vi "globalprogram testen.vi"() -> (2 "Array 2":i32[](array[numeric]), 3 "Numeric 2":i32)   [LabVIEW 2019]
uses:
  <vilib>/myRIO/Common/Instrument Driver Framework/Utilities/typedefs/Analog Scaling Constants.ctl
  <vilib>/myRIO/Common/Instrument Driver Framework/Utilities/typedefs/Analog Scaling Constants List.ctl
  <vilib>/myRIO/Common/Instrument Driver Framework/myRIO v1.0/AO/typedefs/AO Channels Enum.ctl
  <vilib>/myRIO/Common/Instrument Driver Framework/myRIO v1.0/AO/typedefs/AO Channels List.ctl
  <vilib>/myRIO/Common/Instrument Driver Framework/Utilities/typedefs/Generic FPGA Reference.ctl
  <vilib>/myRIO/Common/Instrument Driver Framework/Utilities/typedefs/myRIO v1.0 Reference.ctl
  <vilib>/myRIO/Common/Instrument Driver Framework/Utilities/typedefs/Hardware Version Enum.ctl
  <vilib>/myRIO/Common/Instrument Driver Framework/Utilities/typedefs/myRIO Generic Hardware Reference.ctl
  <vilib>/myRIO/Instrument Drivers/Onboard IO/AO/typedefs/AO Reference.ctl
  <vilib>/myRIO/Instrument Drivers/Onboard IO/AO/AO.lvlib
  <vilib>/myRIO/Instrument Drivers/Onboard IO/AO/vis/Write.vi
  <vilib>/userDefined/High Color/nirio_resource_hc.ctl
  <vilib>/myRIO/Common/Instrument Driver Framework/myRIO v1.0/AO/vis/myRIO v1.1 Open AO.vi
  <vilib>/myRIO/Instrument Drivers/Onboard IO/AO/vis/myRIO AO Open.xnode
  <vilib>/myRIO/Common/Instrument Driver Framework/Utilities/vis/Is FPGA Ref Available.vi
  <vilib>/myRIO/Express VI/Onboard IO/AO/AO Express VI.xnode
  <vilib>/myRIO/Common/Instrument Driver Framework/myRIO v1.0/DIO/typedefs/DIO Channels Enum.ctl
  <vilib>/myRIO/Common/Instrument Driver Framework/myRIO v1.0/DIO/typedefs/DIO Channels List.ctl
  <vilib>/myRIO/Instrument Drivers/Onboard IO/DIO/typedefs/DIO Reference.ctl
  <vilib>/myRIO/Instrument Drivers/Onboard IO/DIO/DIO.lvlib
  <vilib>/myRIO/Instrument Drivers/Onboard IO/DIO/vis/myRIO DIO Open.xnode
  <vilib>/myRIO/Common/Instrument Driver Framework/myRIO v1.0/DIO/vis/myRIO v1.1 Open DIO.vi
  <vilib>/myRIO/Instrument Drivers/Onboard IO/DIO/vis/Write.vi
  <vilib>/myRIO/Express VI/Onboard IO/DO/DO Express VI.xnode
  <vilib>/myRIO/Express VI/Onboard IO/DI/DI Express VI.xnode
  <vilib>/myRIO/Instrument Drivers/Onboard IO/DIO/vis/Read.vi
  Global.vi
  <vilib>/myRIO/Express VI/Onboard IO/AI/AI Express VI.xnode
  <vilib>/myRIO/Instrument Drivers/Onboard IO/AI/typedefs/AI Reference.ctl
  <vilib>/myRIO/Instrument Drivers/Onboard IO/AI/AI.lvlib
  <vilib>/myRIO/Common/Instrument Driver Framework/myRIO v1.0/AI/typedefs/AI Channels List.ctl
  <vilib>/myRIO/Common/Instrument Driver Framework/myRIO v1.0/AI/typedefs/AI Channels Enum.ctl
  <vilib>/myRIO/Instrument Drivers/Onboard IO/AI/vis/Read.vi
  <vilib>/myRIO/Instrument Drivers/Onboard IO/AI/vis/myRIO AI Open.xnode
  <vilib>/myRIO/Common/Instrument Driver Framework/myRIO v1.0/AI/vis/myRIO v1.1 Open AI.vi
panel:
  in  "MANUEEL":bool
  in  "STOP":bool
  in  "tijdsinterval 8":dbl
  in  "tijdsinterval 7":dbl
  in  "tijdsinterval 6":dbl
  in  "tijdsinterval 5":dbl
  in  "tijdsinterval 4":dbl
  in  "tijdsinterval 3":dbl
  in  "tijdsinterval 2":dbl
  out "A/DIO1 (Pin 13)":bool
  in  "stoppen":bool
  in  "rechts draaien achteruit":bool
  in  "links draaien achteruit":bool
  out "appended array":dbl[](array[numeric])
  in  "snelheid":dbl
  in  "rechts draaien":bool
  in  "links draaien":bool
  in  "achterwaarts":bool
  in  "voorwaarts":bool
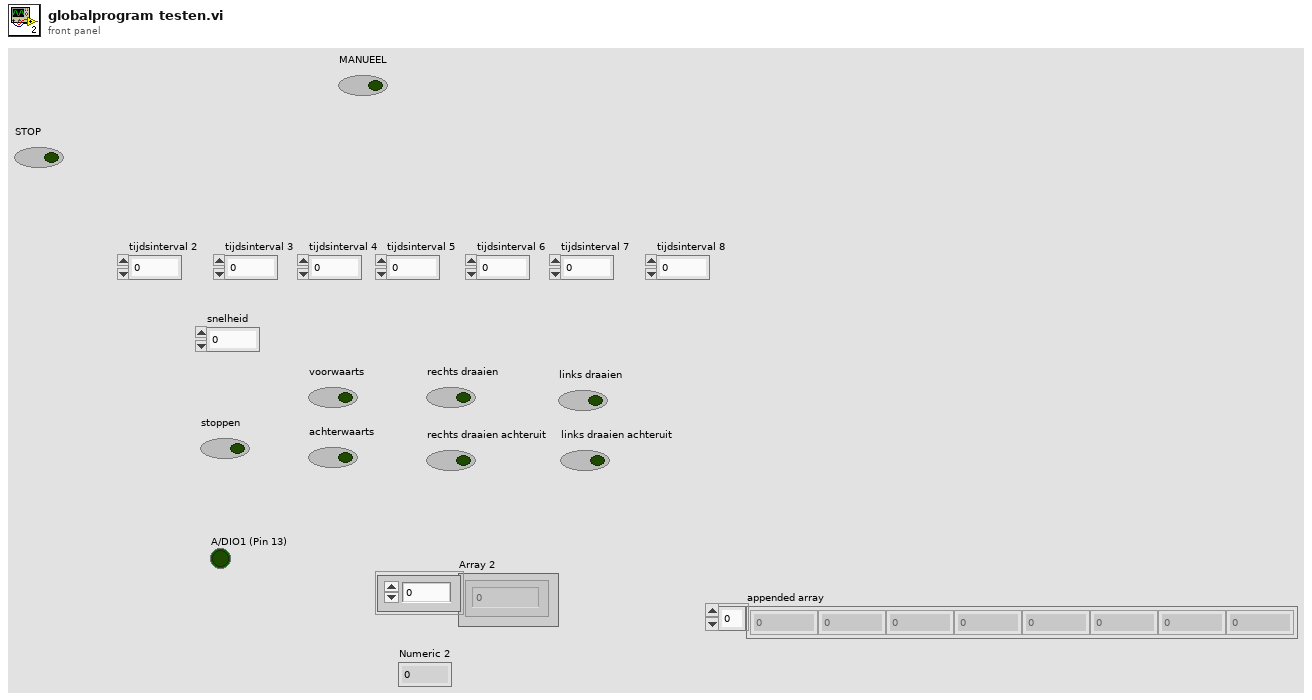
[diagram p1: front panel]
types:
  T1 = typedef "DIO.lvlib/DIO Reference.ctl" = cluster{"myRIO Reference":T2, "DIO Channels List":T6}
  T2 = typedef "myRIO Generic Hardware Reference.ctl" = cluster{"myRIO Model":T3, "myRIO Hardware Reference":T4}
  T3 = typedef "Hardware Version Enum.ctl" = enum16{"Unknown", "myRIO-1900", "myRIO-1950", "roboRIO", "NI ELVIS RIO CM", "ELVIS III"}
  T4 = typedef "myRIO v1.0 Reference.ctl" = cluster{"Generic FPGA Reference":T5, "Allow multiple opens":bool}
  T5 = typedef "Generic FPGA Reference.ctl" = refnum<k20>
  T6 = typedef "DIO Channels List.ctl" = T7[]
  T7 = typedef "DIO Channels Enum.ctl" = enum16{"Not Connected", "C/DIO0", "C/DIO1", "C/DIO2", "C/DIO3", "C/DIO4", "C/DIO5", "C/DIO6", "C/DIO7", "A/DIO0", "A/DIO1", "A/DIO2", "A/DIO3", "A/DIO4", "A/DIO5", "A/DIO6", "A/DIO7", "A/DIO8", "A/DIO9", "A/DIO10", "A/DIO11", "A/DIO12", "A/DIO13", "A/DIO14", "A/DIO15", "A/DIO16", "A/DIO17", "A/DIO18", "A/DIO19", "B/DIO0", "B/DIO1", "B/DIO2", "B/DIO3", "B/DIO4", "B/DIO5", "B/DIO6", "B/DIO7", "B/DIO8", "B/DIO9", "B/DIO10", "B/DIO11", "B/DIO12", "B/DIO13", "B/DIO14", "B/DIO15", "B/DIO16", "B/DIO17", "B/DIO18", "B/DIO19", "LED0", "LED1", "LED2", "LED3", "Button0", "DIO/DIO0", "DIO/DIO1", "DIO/DIO2", "DIO/DIO3", "DIO/DIO4", "DIO/DIO5", "DIO/DIO6", "DIO/DIO7", "DIO/DIO8", "DIO/DIO9", "SPI/CS0", "SPI/CS1", "SPI/CS2", "SPI/CS3", "LED RADIO (Green)", "LED RADIO (Red)", "LED COMM (Green)", "LED COMM (Red)", "LED MODE (Green)", "LED MODE (Red)"}
  T8 = typedef "nirio_resource_hc.ctl" = tag
  T9 = typedef "AO.lvlib/AO Reference.ctl" = cluster{"myRIO Reference":T2, "AO Channel List":T10, "AO Scaling Constant List":T12}
  T10 = typedef "AO Channels List.ctl" = T11[]
  T11 = typedef "AO Channels Enum.ctl" = enum16{"Not Connected", "AudioOut/Left", "AudioOut/Right", "C/AO0", "C/AO1", "A/AO0", "A/AO1", "B/AO0", "B/AO1"}
  T12 = typedef "Analog Scaling Constants List.ctl" = T13[]
  T13 = typedef "Analog Scaling Constants.ctl" = cluster{"LSB Weight (Volts)":dbl, "Offset (Volts)":dbl, "Signed?":bool}
  T14 = typedef "AI.lvlib/AI Reference.ctl" = cluster{"myRIO Reference":T2, "AI Channels List":T15, "AI Scaling Constants List":T12}
  T15 = typedef "AI Channels List.ctl" = T16[]
  T16 = typedef "AI Channels Enum.ctl" = enum16{"Not Connected", "AudioIn/Left", "AudioIn/Right", "C/AI0", "C/AI1", "A/AI0", "A/AI1", "A/AI2", "A/AI3", "A/AI4", "A/AI5", "A/AI6", "A/AI7", "B/AI0", "B/AI1", "B/AI2", "B/AI3", "B/AI4", "B/AI5", "B/AI6", "B/AI7", "AI/AI0", "AI/AI1", "AI/AI2", "AI/AI3", "A/AI0 (DIFF)", "A/AI1 (DIFF)", "A/AI2 (DIFF)", "A/AI3 (DIFF)", "B/AI0 (DIFF)", "B/AI1 (DIFF)", "B/AI2 (DIFF)", "B/AI3 (DIFF)"}
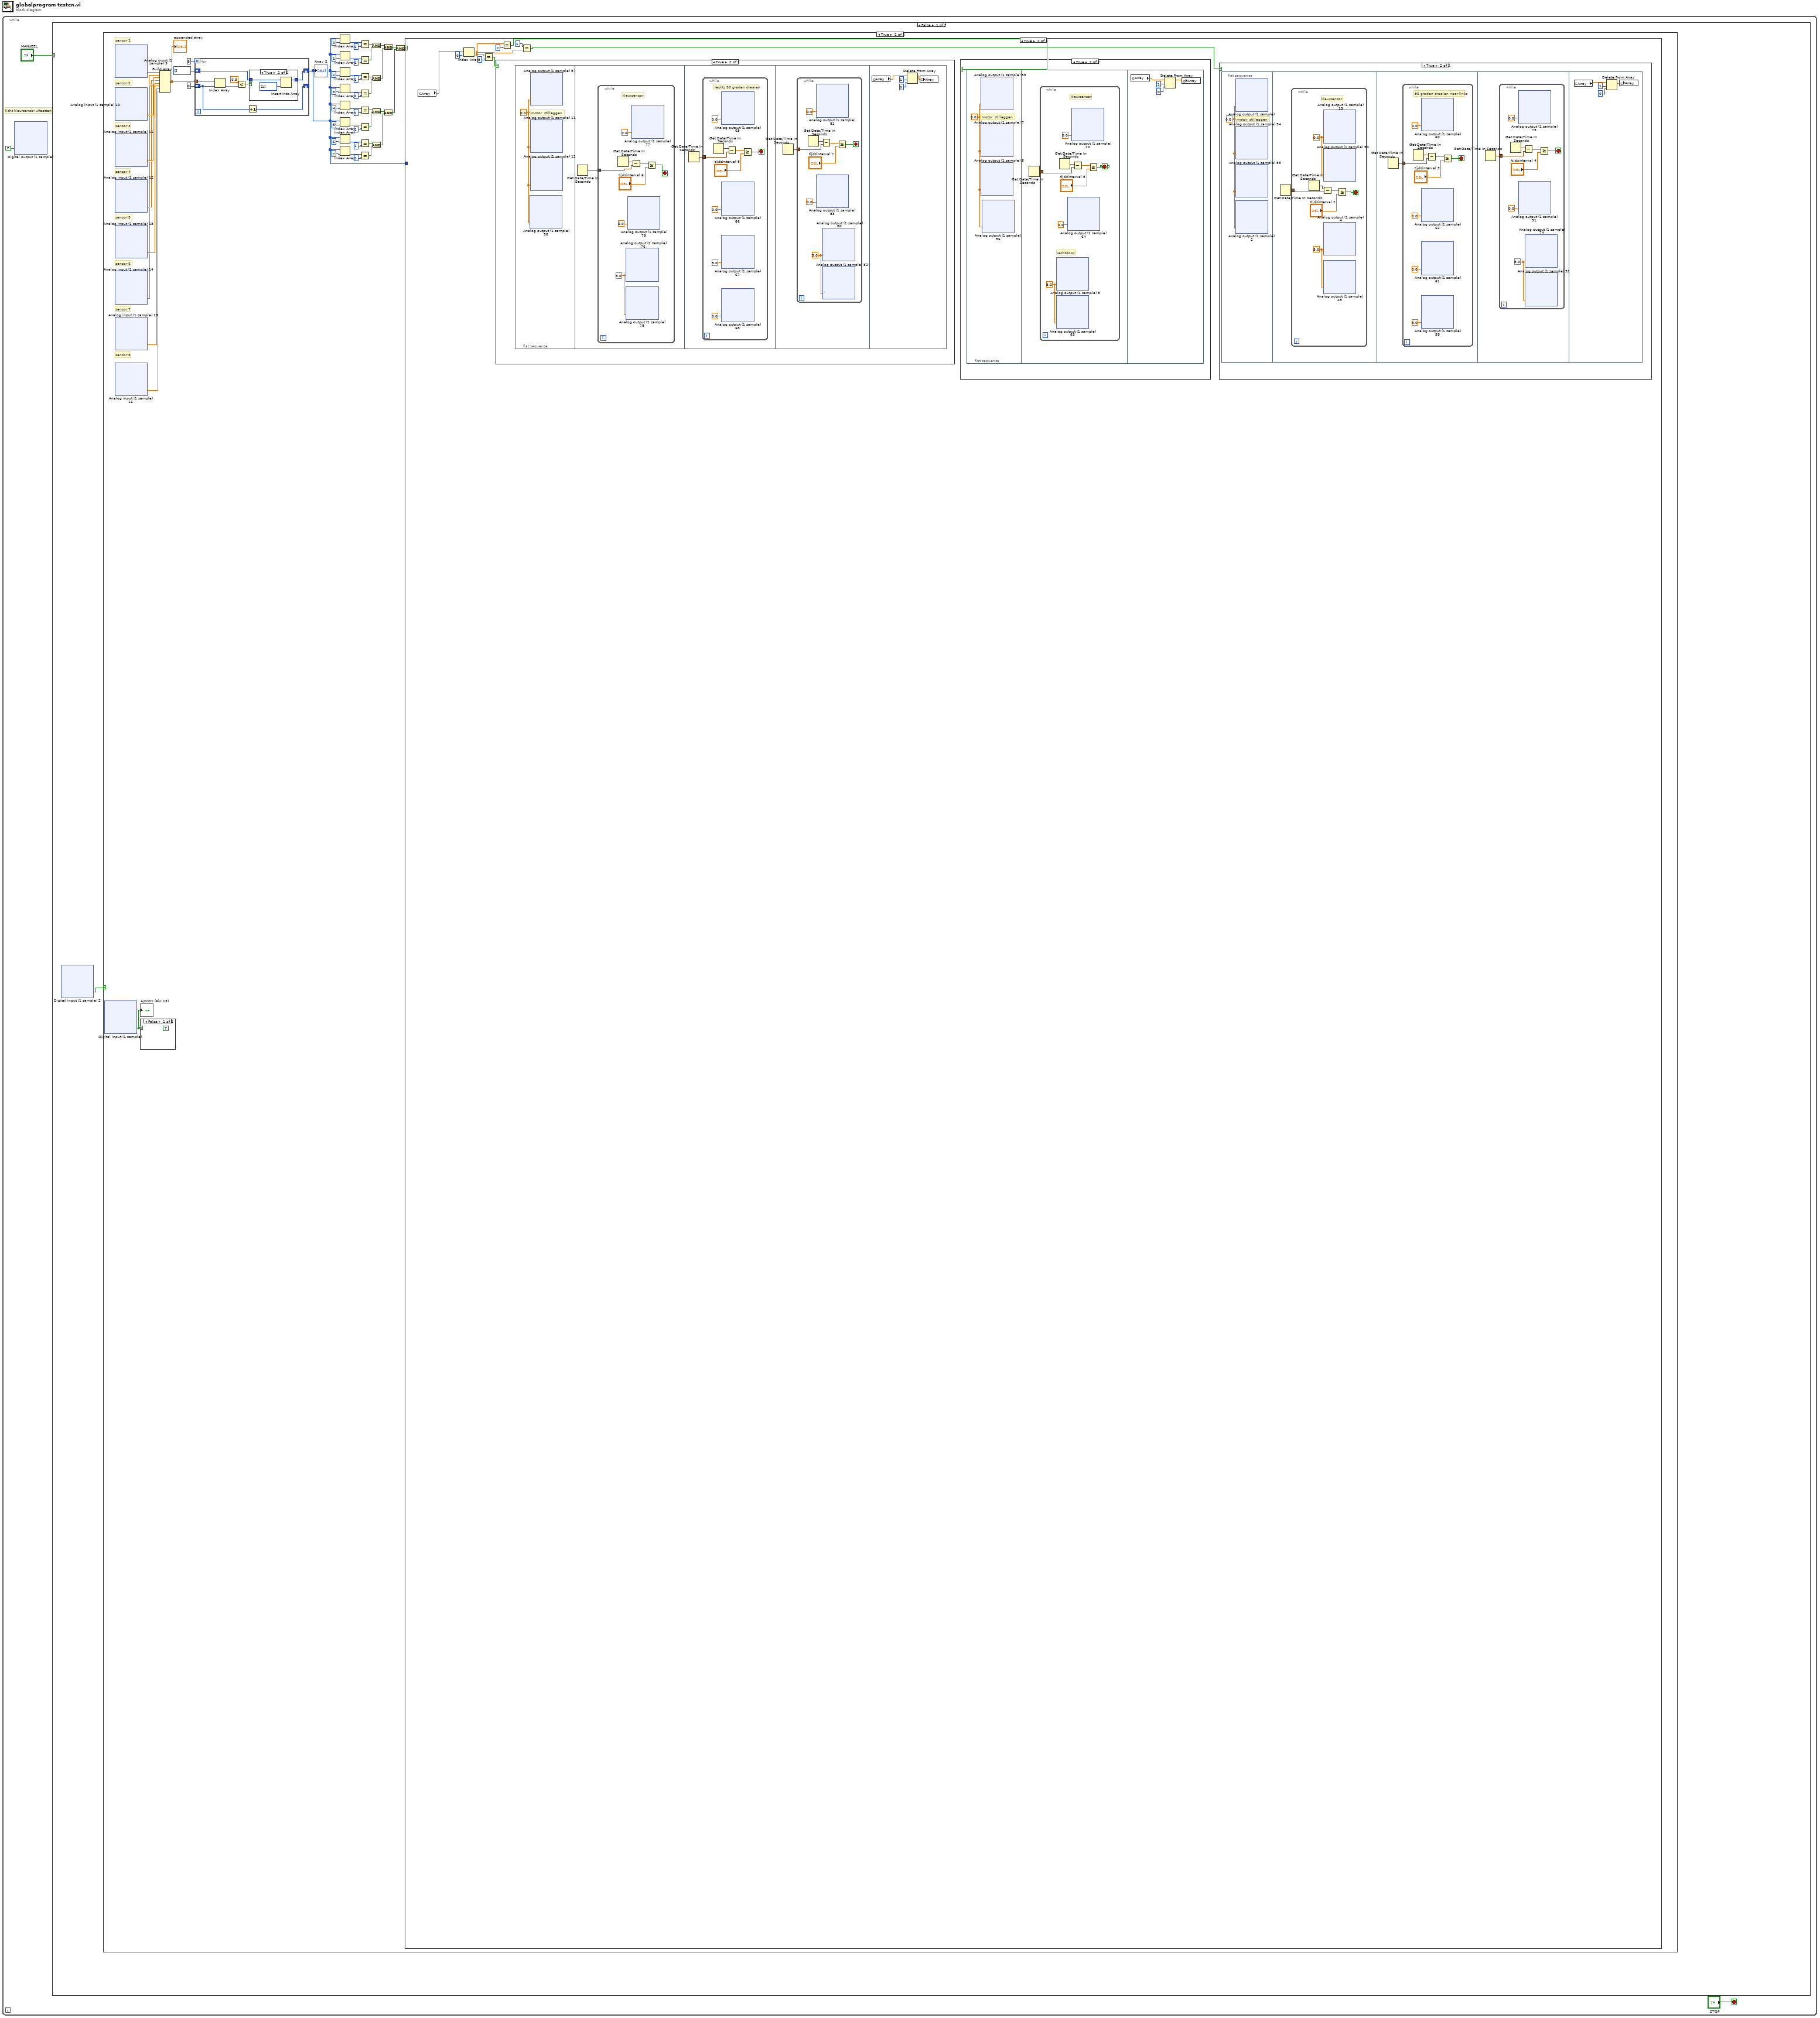
[diagram p0: block diagram]
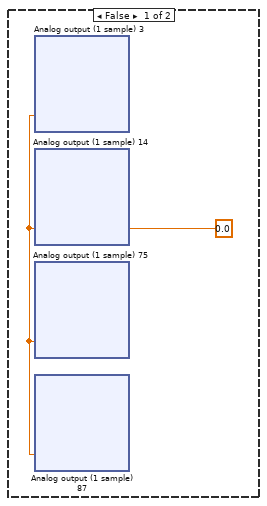
[diagram p2: hidden frame]
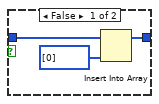
[diagram p3: hidden frame]
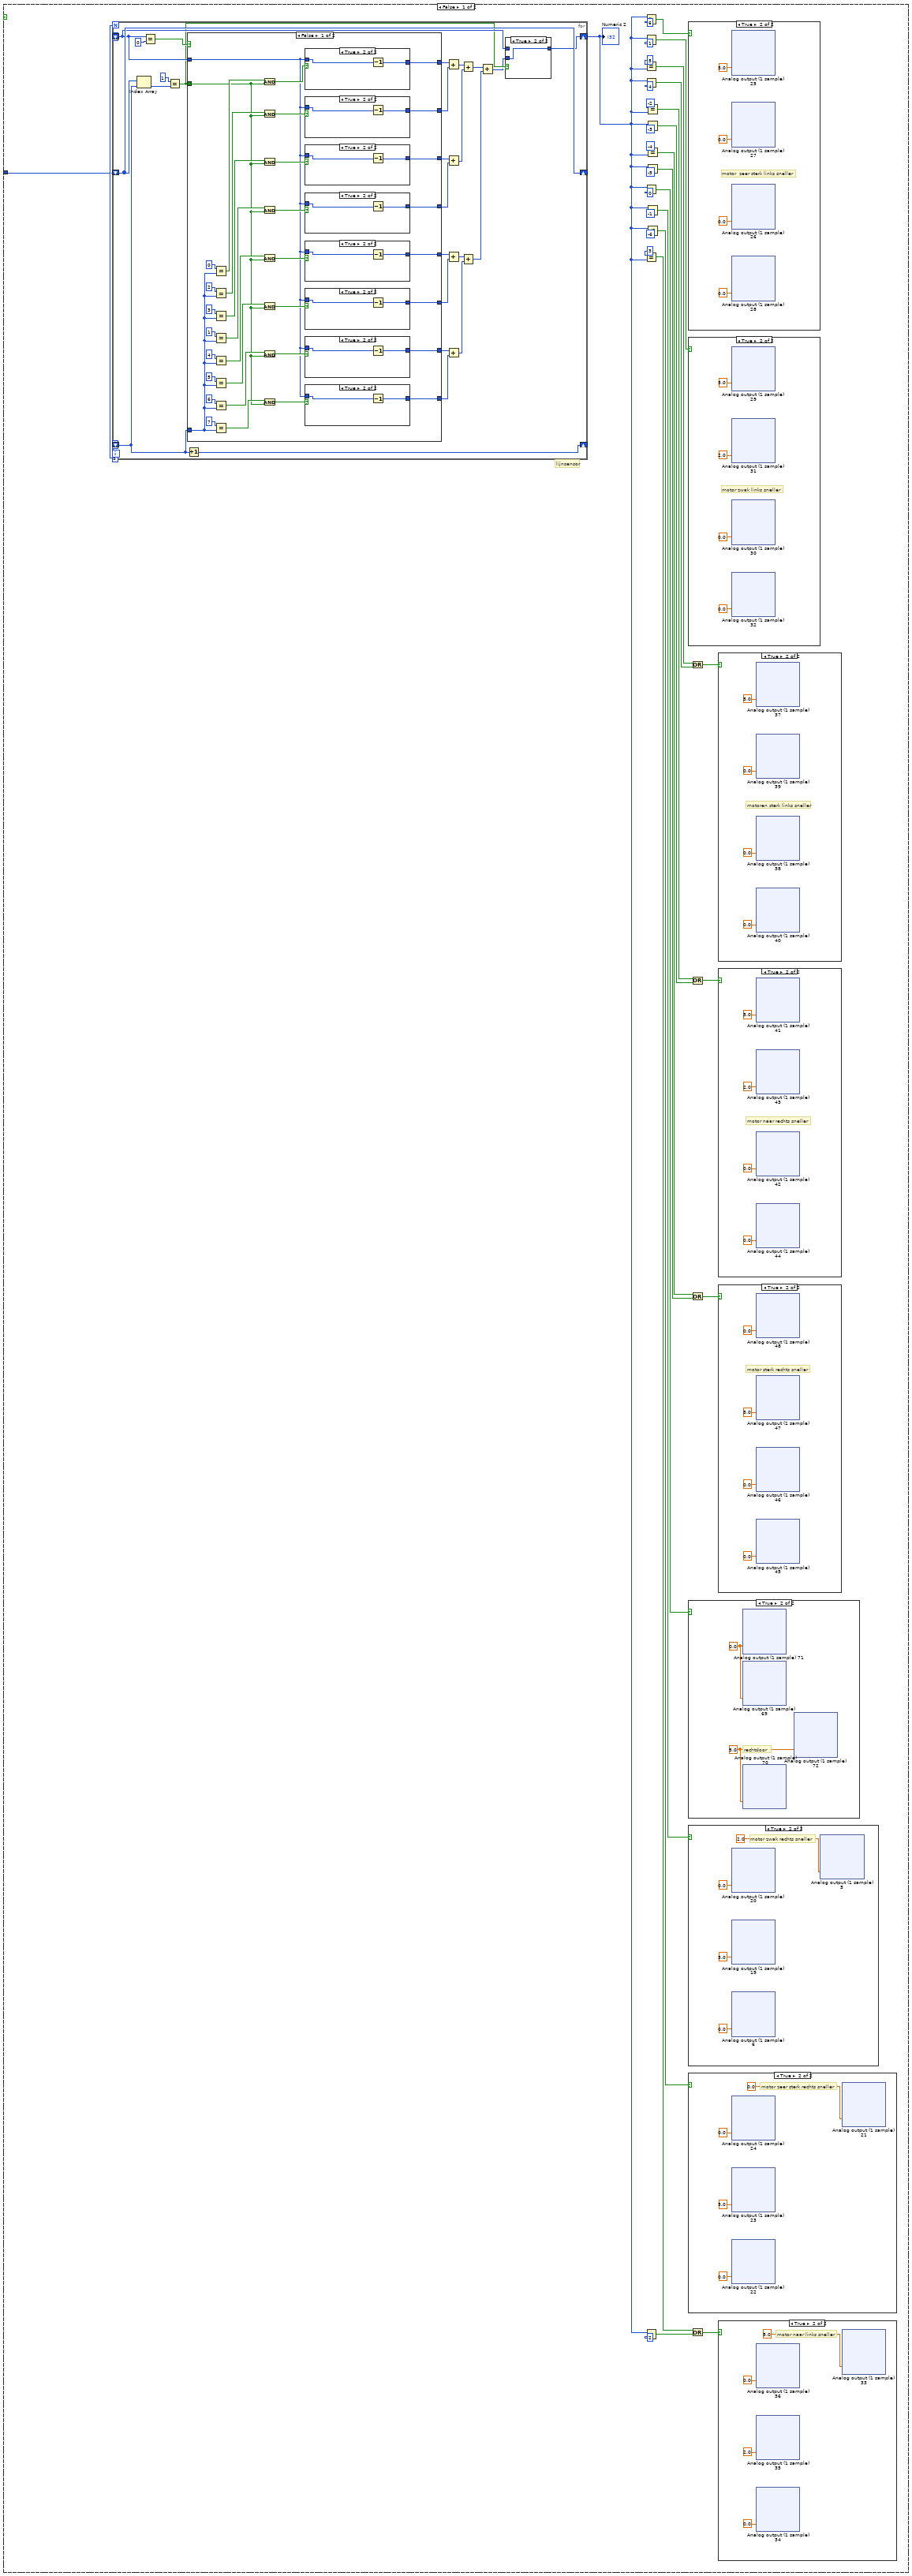
[diagram p4: hidden frame]
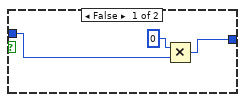
[diagram p15: hidden frame]
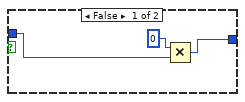
[diagram p16: hidden frame]
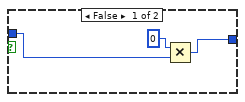
[diagram p17: hidden frame]
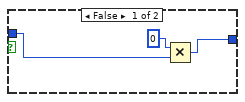
[diagram p18: hidden frame]
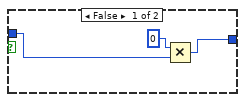
[diagram p19: hidden frame]
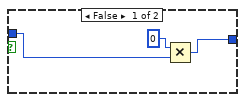
[diagram p20: hidden frame]
diagram:
  n1 = while {
    stop <- "STOP" stop-if-true
    # "licht kleursensor uitzetten"
    n2 = xnode "Digital output (1 sample)"("A/DIO2 (Pin 15)"=FALSE) -> ()  [unwired: 1 in, 1 out]
    n3 = case shown="False" "MANUEEL" {
      frame False {
        n4 = xnode "Digital input (1 sample) 2"() -> ("A/DIO1 (Pin 13)"=w39:bool)  [unwired: 1 in, 1 out]
        n5 = case shown="True" w39 {
          frame False {
            w76 = 0.0
            n6 = xnode "Analog output (1 sample) 3"("A/AO0 (Pin 2)"=w76) -> ()  [unwired: 1 in, 1 out]
            n7 = xnode "Analog output (1 sample) 14"("A/AO1 (Pin 4)"=w76) -> ()  [unwired: 1 in, 1 out]
            n8 = xnode "Analog output (1 sample) 75"("B/AO0 (Pin 2)"=w76) -> ()  [unwired: 1 in, 1 out]
            n9 = xnode "Analog output (1 sample) 87"("B/AO1 (Pin 4)"=w76) -> ()  [unwired: 1 in, 1 out]
          }
          frame True {
            # "sensor 8"
            # "sensor 7"
            # "sensor 6"
            # "sensor 5"
            # "sensor 4"
            # "sensor 3"
            # "sensor 2"
            # "sensor 1"
            n10 = xnode "Analog input (1 sample) 9"() -> ("A/AI3 (Pin 9)"=w233:dbl)  [unwired: 1 in, 1 out]
            n11 = xnode "Analog input (1 sample) 10"() -> ("A/AI2 (Pin 7)"=w232:dbl)  [unwired: 1 in, 1 out]
            n12 = xnode "Analog input (1 sample) 11"() -> ("A/AI1 (Pin 5)"=w231:dbl)  [unwired: 1 in, 1 out]
            n13 = xnode "Analog input (1 sample) 12"() -> ("A/AI0 (Pin 3)"=w230:dbl)  [unwired: 1 in, 1 out]
            n14 = xnode "Analog input (1 sample) 13"() -> ("B/AI3 (Pin 9)"=w229:dbl)  [unwired: 1 in, 1 out]
            n15 = xnode "Analog input (1 sample) 14"() -> ("B/AI2 (Pin 7)"=w228:dbl)  [unwired: 1 in, 1 out]
            n16 = xnode "Analog input (1 sample) 15"() -> ("A/AI1 (Pin 5)"=w227:dbl)  [unwired: 1 in, 1 out]
            n17 = xnode "Analog input (1 sample) 16"() -> ("B/AI0 (Pin 3)"=w226:dbl)  [unwired: 1 in, 1 out]
            n18 = Build Array(w233, w232, w231, w230, w229, w228, w227, w226) -> (w225:dbl[])
            "appended array" <- w225
            n19 = for {
              N: 8 -> [_]
              shift-right: [w579] -> w276
              shift-left: i32[] [] -> [w580]
              shift-right: [w577] -> _
              shift-left: 0 -> [w574]
              tunnel: w225 -> [w575]
              n20 = Index Array(array=w575, index=w574) -> (element=w576:dbl)
              n21 = Less?(x=0.3, y=w576) -> (x < y?=w578:bool)
              n22 = Increment(x=w574) -> (x+1=w577:i32)
              n23 = case shown="True" w578 {
                tunnel: w580 -> [w582 w584]
                tunnel: [w583 w586] -> w579
                frame False {
                  n24 = Insert Into Array(array=w582, new element=i32[] [0]) -> (w583:i32[])  [unwired: 1 in]
                }
                frame True {
                  n25 = Insert Into Array(array=w584, new element=i32[] [1]) -> (w586:i32[])  [unwired: 1 in]
                }
              }
            }
            "Array 2" <- w276
            n26 = Index Array(array=w276, index=0) -> (element=w255:i32)
            n27 = Index Array(array=w276, index=1) -> (element=w234:i32)
            n28 = Index Array(array=w276, index=2) -> (element=w240:i32)
            n29 = Index Array(array=w276, index=3) -> (element=w237:i32)
            n30 = Index Array(array=w276, index=4) -> (element=w243:i32)
            n31 = Index Array(array=w276, index=5) -> (element=w246:i32)
            n32 = Index Array(array=w276, index=6) -> (element=w249:i32)
            n33 = Index Array(array=w276, index=7) -> (element=w252:i32)
            n34 = Equal?(x=w255, y=1) -> (x = y?=w258:bool)
            n35 = Equal?(x=w234, y=1) -> (x = y?=w259:bool)
            n36 = Equal?(x=w240, y=1) -> (x = y?=w260:bool)
            n37 = Equal?(x=w237, y=1) -> (x = y?=w261:bool)
            n38 = Equal?(x=w243, y=1) -> (x = y?=w262:bool)
            n39 = Equal?(x=w246, y=1) -> (x = y?=w263:bool)
            n40 = Equal?(x=w249, y=1) -> (x = y?=w264:bool)
            n41 = Equal?(x=w252, y=1) -> (x = y?=w265:bool)
            n42 = And(x=w258, y=w259) -> (x .and. y?=w266:bool)
            n43 = And(x=w260, y=w261) -> (x .and. y?=w267:bool)
            n44 = And(x=w262, y=w263) -> (x .and. y?=w268:bool)
            n45 = And(x=w264, y=w265) -> (x .and. y?=w269:bool)
            n46 = And(x=w266, y=w267) -> (x .and. y?=w270:bool)
            n47 = And(x=w268, y=w269) -> (x .and. y?=w271:bool)
            n48 = And(x=w270, y=w271) -> (x .and. y?=w272:bool)
            n49 = case shown="True" w272 {
              tunnel: w276 -> [w590 _]
              frame False {
                # "lijnsensor"
                n50 = for {
                  N: 8 -> [_]
                  shift-right: [w1998] -> _
                  shift-left: 0 -> [w2012]
                  shift-right: [w1990] -> w587
                  shift-left: 0 -> [w1991]
                  shift-right: [w2003] -> _
                  shift-left: w590 -> [w2003]
                  n51 = Index Array(array=w2003, index=w2012) -> (element=w2002:i32)
                  n52 = Equal?(x=w1991, y=0) -> (x = y?=w1999:bool)
                  n53 = Equal?(x=1, y=w2002) -> (x = y?=w1989:bool)
                  n54 = Increment(x=w2012) -> (x+1=w1998:i32)
                  n55 = case shown="False" w1999 {
                    tunnel: w2012 -> [w2022 w2108]
                    tunnel: [w2016 w2107] -> w2011
                    tunnel: [w2023 w2106] -> w2010
                    tunnel: [w2024 w2105] -> w2009
                    tunnel: [w2025 w2104] -> w2008
                    tunnel: w1991 -> [w2015 w2103]
                    tunnel: w1989 -> [w2021 w2094]
                    tunnel: [w2019 w2093] -> w1997
                    tunnel: [w2020 w2092] -> w1996
                    tunnel: [w2017 w2091] -> w1994
                    tunnel: [w2018 w2090] -> w1993
                    frame False {
                      n56 = Equal?(x=0, y=w2022) -> (x = y?=w2042:bool)
                      n57 = Equal?(x=2, y=w2022) -> (x = y?=w2048:bool)
                      n58 = Equal?(x=3, y=w2022) -> (x = y?=w2049:bool)
                      n59 = Equal?(x=1, y=w2022) -> (x = y?=w2034:bool)
                      n60 = Equal?(x=4, y=w2022) -> (x = y?=w2046:bool)
                      n61 = Equal?(x=5, y=w2022) -> (x = y?=w2047:bool)
                      n62 = Equal?(x=6, y=w2022) -> (x = y?=w2045:bool)
                      n63 = Equal?(x=7, y=w2022) -> (x = y?=w2044:bool)
                      n64 = And(x=w2042, y=w2021) -> (x .and. y?=w2026:bool)
                      n65 = And(x=w2048, y=w2021) -> (x .and. y?=w2028:bool)
                      n66 = And(x=w2049, y=w2021) -> (x .and. y?=w2029:bool)
                      n67 = And(x=w2034, y=w2021) -> (x .and. y?=w2027:bool)
                      n68 = And(x=w2046, y=w2021) -> (x .and. y?=w2030:bool)
                      n69 = And(x=w2047, y=w2021) -> (x .and. y?=w2031:bool)
                      n70 = And(x=w2045, y=w2021) -> (x .and. y?=w2032:bool)
                      n71 = And(x=w2044, y=w2021) -> (x .and. y?=w2033:bool)
                      n72 = case shown="True" w2026 {
                        tunnel: [w2051 w2054] -> w2020
                        tunnel: w2015 -> [w2050 w2053]
                        frame False {
                          n73 = Multiply(x=0, y=w2050) -> (x*y=w2051:i32)
                        }
                        frame True {
                          n74 = Decrement(x=w2053) -> (x-1=w2054:i32)
                        }
                      }
                      n75 = case shown="True" w2028 {
                        tunnel: [w2082 w2083] -> w2019
                        tunnel: w2015 -> [w2081 w2084]
                        frame False {
                          n76 = Multiply(x=0, y=w2081) -> (x*y=w2082:i32)
                        }
                        frame True {
                          n77 = Decrement(x=w2084) -> (x-1=w2083:i32)
                        }
                      }
                      n78 = case shown="True" w2029 {
                        tunnel: [w2076 w2079] -> w2018
                        tunnel: w2015 -> [w2075 w2078]
                        frame False {
                          n79 = Multiply(x=0, y=w2075) -> (x*y=w2076:i32)
                        }
                        frame True {
                          n80 = Decrement(x=w2078) -> (x-1=w2079:i32)
                        }
                      }
                      n81 = case shown="True" w2027 {
                        tunnel: [w2086 w2089] -> w2017
                        tunnel: w2015 -> [w2085 w2088]
                        frame False {
                          n82 = Multiply(x=0, y=w2085) -> (x*y=w2086:i32)
                        }
                        frame True {
                          n83 = Decrement(x=w2088) -> (x-1=w2089:i32)
                        }
                      }
                      n84 = case shown="True" w2030 {
                        tunnel: [w2071 w2074] -> w2016
                        tunnel: w2015 -> [w2070 w2073]
                        frame False {
                          n85 = Multiply(x=0, y=w2070) -> (x*y=w2071:i32)
                        }
                        frame True {
                          n86 = Decrement(x=w2073) -> (x-1=w2074:i32)
                        }
                      }
                      n87 = case shown="True" w2031 {
                        tunnel: [w2061 w2064] -> w2023
                        tunnel: w2015 -> [w2060 w2063]
                        frame False {
                          n88 = Multiply(x=0, y=w2060) -> (x*y=w2061:i32)
                        }
                        frame True {
                          n89 = Decrement(x=w2063) -> (x-1=w2064:i32)
                        }
                      }
                      n90 = case shown="True" w2032 {
                        tunnel: [w2066 w2069] -> w2024
                        tunnel: w2015 -> [w2065 w2068]
                        frame False {
                          n91 = Multiply(x=0, y=w2065) -> (x*y=w2066:i32)
                        }
                        frame True {
                          n92 = Decrement(x=w2068) -> (x-1=w2069:i32)
                        }
                      }
                      n93 = case shown="True" w2033 {
                        tunnel: [w2055 w2059] -> w2025
                        tunnel: w2015 -> [w2056 w2058]
                        frame False {
                          n94 = Multiply(x=0, y=w2056) -> (x*y=w2055:i32)
                        }
                        frame True {
                          n95 = Decrement(x=w2058) -> (x-1=w2059:i32)
                        }
                      }
                    }
                    frame True {
                      n96 = Equal?(x=0, y=w2108) -> (x = y?=w2117:bool)
                      n97 = Equal?(x=1, y=w2108) -> (x = y?=w2109:bool)
                      n98 = Equal?(x=2, y=w2108) -> (x = y?=w2123:bool)
                      n99 = Equal?(x=3, y=w2108) -> (x = y?=w2124:bool)
                      n100 = Equal?(x=4, y=w2108) -> (x = y?=w2121:bool)
                      n101 = Equal?(x=5, y=w2108) -> (x = y?=w2122:bool)
                      n102 = Equal?(x=6, y=w2108) -> (x = y?=w2120:bool)
                      n103 = Equal?(x=7, y=w2108) -> (x = y?=w2119:bool)
                      n104 = And(x=w2117, y=w2094) -> (x .and. y?=w2095:bool)
                      n105 = And(x=w2109, y=w2094) -> (x .and. y?=w2096:bool)
                      n106 = And(x=w2123, y=w2094) -> (x .and. y?=w2097:bool)
                      n107 = And(x=w2124, y=w2094) -> (x .and. y?=w2098:bool)
                      n108 = And(x=w2121, y=w2094) -> (x .and. y?=w2099:bool)
                      n109 = And(x=w2122, y=w2094) -> (x .and. y?=w2100:bool)
                      n110 = And(x=w2120, y=w2094) -> (x .and. y?=w2101:bool)
                      n111 = And(x=w2119, y=w2094) -> (x .and. y?=w2102:bool)
                      n112 = case shown="True" w2095 {
                        tunnel: w2103 -> [w2125 w2129]
                        tunnel: [w2126 w2128] -> w2092
                        frame False {
                          n113 = Multiply(x=0, y=w2125) -> (x*y=w2126:i32)
                        }
                        frame True {
                          n114 = Add(x=7, y=w2129) -> (x+y=w2128:i32)
                        }
                      }
                      n115 = case shown="True" w2096 {
                        tunnel: w2103 -> [w2165 w2168]
                        tunnel: [w2166 w2169] -> w2093
                        frame False {
                          n116 = Multiply(x=0, y=w2165) -> (x*y=w2166:i32)
                        }
                        frame True {
                          n117 = Add(x=5, y=w2168) -> (x+y=w2169:i32)
                        }
                      }
                      n118 = case shown="True" w2097 {
                        tunnel: w2103 -> [w2159 w2163]
                        tunnel: [w2160 w2162] -> w2090
                        frame False {
                          n119 = Multiply(x=0, y=w2159) -> (x*y=w2160:i32)
                        }
                        frame True {
                          n120 = Add(x=3, y=w2163) -> (x+y=w2162:i32)
                        }
                      }
                      n121 = case shown="True" w2098 {
                        tunnel: w2103 -> [w2155 w2158]
                        tunnel: [w2154 w2157] -> w2091
                        frame False {
                          n122 = Multiply(x=0, y=w2155) -> (x*y=w2154:i32)
                        }
                        frame True {
                          n123 = Increment(x=w2158) -> (x+1=w2157:i32)
                        }
                      }
                      n124 = case shown="True" w2099 {
                        tunnel: w2103 -> [w2149 w2153]
                        tunnel: [w2150 w2152] -> w2107
                        frame False {
                          n125 = Multiply(x=0, y=w2149) -> (x*y=w2150:i32)
                        }
                        frame True {
                          n126 = Decrement(x=w2153) -> (x-1=w2152:i32)
                        }
                      }
                      n127 = case shown="True" w2100 {
                        tunnel: w2103 -> [w2138 w2140]
                        tunnel: [w2137 w2142] -> w2106
                        frame False {
                          n128 = Multiply(x=0, y=w2138) -> (x*y=w2137:i32)
                        }
                        frame True {
                          n129 = Subtract(x=w2140, y=3) -> (x-y=w2142:i32)
                        }
                      }
                      n130 = case shown="True" w2101 {
                        tunnel: w2103 -> [w2144 w2146]
                        tunnel: [w2143 w2147] -> w2105
                        frame False {
                          n131 = Multiply(x=0, y=w2144) -> (x*y=w2143:i32)
                        }
                        frame True {
                          n132 = Subtract(x=w2146, y=5) -> (x-y=w2147:i32)
                        }
                      }
                      n133 = case shown="True" w2102 {
                        tunnel: w2103 -> [w2131 w2134]
                        tunnel: [w2132 w2135] -> w2104
                        frame False {
                          n134 = Multiply(x=0, y=w2131) -> (x*y=w2132:i32)
                        }
                        frame True {
                          n135 = Subtract(x=w2134, y=7) -> (x-y=w2135:i32)
                        }
                      }
                    }
                  }
                  n136 = Add(x=w1996, y=w1997) -> (x+y=w1995:i32)
                  n137 = Add(x=w1993, y=w1994) -> (x+y=w1992:i32)
                  n138 = Add(x=w2011, y=w2010) -> (x+y=w2006:i32)
                  n139 = Add(x=w2009, y=w2008) -> (x+y=w2007:i32)
                  n140 = Add(x=w1995, y=w1992) -> (x+y=w2005:i32)
                  n141 = Add(x=w2006, y=w2007) -> (x+y=w2004:i32)
                  n142 = Add(x=w2005, y=w2004) -> (x+y=w1988:i32)
                  n143 = case shown="True" w1989 {
                    tunnel: w1991 -> [w2013 _]
                    tunnel: [w2013 w2014] -> w1990
                    tunnel: w1988 -> [_ w2014]
                    frame False {
                    }
                    frame True {
                    }
                  }
                }
                "Numeric 2" <- w587
                n144 = Greater Or Equal?(x=w587, y=6) -> (x >= y?=w616:bool)
                n145 = Equal?(x=w587, y=1) -> (x = y?=w617:bool)
                n146 = Equal?(x=5, y=w587) -> (x = y?=w611:bool)
                n147 = Equal?(x=w587, y=4) -> (x = y?=w612:bool)
                n148 = Equal?(x=w587, y=0) -> (x = y?=w588:bool)
                n149 = Equal?(x=3, y=w587) -> (x = y?=w607:bool)
                n150 = Equal?(x=w587, y=2) -> (x = y?=w608:bool)
                n151 = Equal?(x=-2, y=w587) -> (x = y?=w601:bool)
                n152 = Equal?(x=w587, y=-3) -> (x = y?=w602:bool)
                n153 = Equal?(x=-4, y=w587) -> (x = y?=w597:bool)
                n154 = Equal?(x=w587, y=-5) -> (x = y?=w598:bool)
                n155 = Equal?(x=w587, y=-1) -> (x = y?=w595:bool)
                n156 = Less Or Equal?(x=w587, y=-6) -> (x <= y?=w593:bool)
                n157 = case shown="True" w616 {
                  frame False {
                  }
                  frame True {
                    # "motor  zeer sterk links sneller"
                    n158 = xnode "Analog output (1 sample) 25"("A/AO0 (Pin 2)"=5.0) -> ()  [unwired: 1 in, 1 out]
                    n159 = xnode "Analog output (1 sample) 27"("B/AO0 (Pin 2)"=0.0) -> ()  [unwired: 1 in, 1 out]
                    n160 = xnode "Analog output (1 sample) 26"("A/AO1 (Pin 4)"=0.0) -> ()  [unwired: 1 in, 1 out]
                    n161 = xnode "Analog output (1 sample) 28"("B/AO1 (Pin 4)"=0.0) -> ()  [unwired: 1 in, 1 out]
                  }
                }
                n162 = case shown="True" w617 {
                  frame False {
                  }
                  frame True {
                    # "motor zwak links sneller"
                    n163 = xnode "Analog output (1 sample) 29"("A/AO0 (Pin 2)"=5.0) -> ()  [unwired: 1 in, 1 out]
                    n164 = xnode "Analog output (1 sample) 31"("B/AO0 (Pin 2)"=2.0) -> ()  [unwired: 1 in, 1 out]
                    n165 = xnode "Analog output (1 sample) 30"("A/AO1 (Pin 4)"=0.0) -> ()  [unwired: 1 in, 1 out]
                    n166 = xnode "Analog output (1 sample) 32"("B/AO1 (Pin 4)"=0.0) -> ()  [unwired: 1 in, 1 out]
                  }
                }
                n167 = case shown="True" w588 {
                  frame False {
                  }
                  frame True {
                    w623 = 0.0
                    w622 = 5.0
                    # "rechtdoor"
                    n168 = xnode "Analog output (1 sample) 71"("A/AO1 (Pin 4)"=w623) -> ()  [unwired: 1 in, 1 out]
                    n169 = xnode "Analog output (1 sample) 69"("B/AO1 (Pin 4)"=w623) -> ()  [unwired: 1 in, 1 out]
                    n170 = xnode "Analog output (1 sample) 70"("B/AO0 (Pin 2)"=w622) -> ()  [unwired: 1 in, 1 out]
                    n171 = xnode "Analog output (1 sample) 72"("A/AO0 (Pin 2)"=w622) -> ()  [unwired: 1 in, 1 out]
                  }
                }
                n172 = case shown="True" w595 {
                  frame False {
                  }
                  frame True {
                    # "motor zwak rechts sneller"
                    n173 = xnode "Analog output (1 sample) 20"("B/AO1 (Pin 4)"=0.0) -> ()  [unwired: 1 in, 1 out]
                    n174 = xnode "Analog output (1 sample) 19"("B/AO0 (Pin 2)"=5.0) -> ()  [unwired: 1 in, 1 out]
                    n175 = xnode "Analog output (1 sample) 6"("A/AO1 (Pin 4)"=0.0) -> ()  [unwired: 1 in, 1 out]
                    n176 = xnode "Analog output (1 sample) 5"("A/AO0 (Pin 2)"=2.0) -> ()  [unwired: 1 in, 1 out]
                  }
                }
                n177 = case shown="True" w593 {
                  frame False {
                  }
                  frame True {
                    # "motor zeer sterk rechts sneller"
                    n178 = xnode "Analog output (1 sample) 24"("B/AO1 (Pin 4)"=0.0) -> ()  [unwired: 1 in, 1 out]
                    n179 = xnode "Analog output (1 sample) 23"("B/AO0 (Pin 2)"=5.0) -> ()  [unwired: 1 in, 1 out]
                    n180 = xnode "Analog output (1 sample) 22"("A/AO1 (Pin 4)"=0.0) -> ()  [unwired: 1 in, 1 out]
                    n181 = xnode "Analog output (1 sample) 21"("A/AO0 (Pin 2)"=0.0) -> ()  [unwired: 1 in, 1 out]
                  }
                }
                n182 = Or(x=w611, y=w612) -> (x .or. y?=w613:bool)
                n183 = Or(x=w601, y=w602) -> (x .or. y?=w594:bool)
                n184 = Or(x=w597, y=w598) -> (x .or. y?=w591:bool)
                n185 = Or(x=w607, y=w608) -> (x .or. y?=w605:bool)
                n186 = case shown="True" w613 {
                  frame False {
                  }
                  frame True {
                    # "motoren sterk links sneller"
                    n187 = xnode "Analog output (1 sample) 37"("A/AO0 (Pin 2)"=5.0) -> ()  [unwired: 1 in, 1 out]
                    n188 = xnode "Analog output (1 sample) 39"("B/AO0 (Pin 2)"=0.0) -> ()  [unwired: 1 in, 1 out]
                    n189 = xnode "Analog output (1 sample) 38"("A/AO1 (Pin 4)"=0.0) -> ()  [unwired: 1 in, 1 out]
                    n190 = xnode "Analog output (1 sample) 40"("B/AO1 (Pin 4)"=0.0) -> ()  [unwired: 1 in, 1 out]
                  }
                }
                n191 = case shown="True" w594 {
                  frame False {
                  }
                  frame True {
                    # "motor naar rechts sneller"
                    n192 = xnode "Analog output (1 sample) 41"("A/AO0 (Pin 2)"=5.0) -> ()  [unwired: 1 in, 1 out]
                    n193 = xnode "Analog output (1 sample) 43"("B/AO0 (Pin 2)"=2.0) -> ()  [unwired: 1 in, 1 out]
                    n194 = xnode "Analog output (1 sample) 42"("A/AO1 (Pin 4)"=0.0) -> ()  [unwired: 1 in, 1 out]
                    n195 = xnode "Analog output (1 sample) 44"("B/AO1 (Pin 4)"=0.0) -> ()  [unwired: 1 in, 1 out]
                  }
                }
                n196 = case shown="True" w591 {
                  frame False {
                  }
                  frame True {
                    # "motor sterk rechts sneller"
                    n197 = xnode "Analog output (1 sample) 48"("B/AO1 (Pin 4)"=0.0) -> ()  [unwired: 1 in, 1 out]
                    n198 = xnode "Analog output (1 sample) 47"("B/AO0 (Pin 2)"=5.0) -> ()  [unwired: 1 in, 1 out]
                    n199 = xnode "Analog output (1 sample) 46"("A/AO1 (Pin 4)"=0.0) -> ()  [unwired: 1 in, 1 out]
                    n200 = xnode "Analog output (1 sample) 45"("A/AO0 (Pin 2)"=0.0) -> ()  [unwired: 1 in, 1 out]
                  }
                }
                n201 = case shown="True" w605 {
                  frame False {
                  }
                  frame True {
                    # "motor naar links sneller"
                    n202 = xnode "Analog output (1 sample) 36"("B/AO1 (Pin 4)"=0.0) -> ()  [unwired: 1 in, 1 out]
                    n203 = xnode "Analog output (1 sample) 35"("B/AO0 (Pin 2)"=2.0) -> ()  [unwired: 1 in, 1 out]
                    n204 = xnode "Analog output (1 sample) 34"("A/AO1 (Pin 4)"=0.0) -> ()  [unwired: 1 in, 1 out]
                    n205 = xnode "Analog output (1 sample) 33"("A/AO0 (Pin 2)"=5.0) -> ()  [unwired: 1 in, 1 out]
                  }
                }
              }
              frame True {
                n206 = global read "Global.vi" "Array"() -> (w2171:dbl[])
                n207 = Index Array(array=w2171, index=0) -> (element=w2175:dbl)
                n208 = Equal?(x=w2175, y=3) -> (x = y?=w2177:bool)
                n209 = case shown="True" w2177 {
                  frame False {
                  }
                  frame True {
                    n210 = flat-sequence {
                      frame #0 {
                        w2180 = 0.0
                        # "motor  stilleggen"
                        n211 = xnode "Analog output (1 sample) 58"("B/AO1 (Pin 4)"=w2180) -> ()  [unwired: 1 in, 1 out]
                        n212 = xnode "Analog output (1 sample) 57"("A/AO1 (Pin 4)"=w2180) -> ()  [unwired: 1 in, 1 out]
                        n213 = xnode "Analog output (1 sample) 11"("B/AO0 (Pin 2)"=w2180) -> ()  [unwired: 1 in, 1 out]
                        n214 = xnode "Analog output (1 sample) 12"("A/AO0 (Pin 2)"=w2180) -> ()  [unwired: 1 in, 1 out]
                      }
                      frame #1 {
                        n215 = Get Date/Time In Seconds() -> (seconds since 1Jan1904=w2329:timestamp)
                        n216 = while {
                          tunnel: w2329 -> [w2334]
                          stop <- w2330 stop-if-true
                          w2332 = 5.0
                          # "kleursensor"
                          n217 = Get Date/Time In Seconds() -> (seconds since 1Jan1904=w2337:timestamp)
                          n218 = xnode "Analog output (1 sample) 76"("A/AO0 (Pin 2)"=w2332) -> ()  [unwired: 1 in, 1 out]
                          n219 = xnode "Analog output (1 sample) 78"("B/AO0 (Pin 2)"=w2332) -> ()  [unwired: 1 in, 1 out]
                          n220 = xnode "Analog output (1 sample) 79"("B/AO1 (Pin 4)"=0.0) -> ()  [unwired: 1 in, 1 out]
                          n221 = Subtract(x=w2337, y=w2334) -> (x-y=w2335:dbl)
                          n222 = xnode "Analog output (1 sample) 77"("A/AO1 (Pin 4)"=0.0) -> ()  [unwired: 1 in, 1 out]
                          n223 = Greater Or Equal?(x=w2335, y="tijdsinterval 6") -> (x >= y?=w2330:bool)
                        }
                      }
                      frame #2 {
                        n224 = Get Date/Time In Seconds() -> (seconds since 1Jan1904=w2486:timestamp)
                        n225 = while {
                          tunnel: w2486 -> [w2488]
                          stop <- w2489 stop-if-true
                          # "rechts 90 graden draaien"
                          n226 = Get Date/Time In Seconds() -> (seconds since 1Jan1904=w2492:timestamp)
                          n227 = xnode "Analog output (1 sample) 65"("A/AO0 (Pin 2)"=0.0) -> ()  [unwired: 1 in, 1 out]
                          n228 = xnode "Analog output (1 sample) 66"("A/AO1 (Pin 4)"=0.0) -> ()  [unwired: 1 in, 1 out]
                          n229 = xnode "Analog output (1 sample) 67"("B/AO0 (Pin 2)"=5.0) -> ()  [unwired: 1 in, 1 out]
                          n230 = xnode "Analog output (1 sample) 68"("B/AO1 (Pin 4)"=0.0) -> ()  [unwired: 1 in, 1 out]
                          n231 = Subtract(x=w2492, y=w2488) -> (x-y=w2490:dbl)
                          n232 = Greater Or Equal?(x=w2490, y="tijdsinterval 8") -> (x >= y?=w2489:bool)
                        }
                      }
                      frame #3 {
                        n233 = Get Date/Time In Seconds() -> (seconds since 1Jan1904=w2644:timestamp)
                        n234 = while {
                          tunnel: w2644 -> [w2646]
                          stop <- w2645 stop-if-true
                          w2651 = 5.0
                          n235 = Get Date/Time In Seconds() -> (seconds since 1Jan1904=w2649:timestamp)
                          n236 = xnode "Analog output (1 sample) 81"("A/AO1 (Pin 4)"=0.0) -> ()  [unwired: 1 in, 1 out]
                          n237 = xnode "Analog output (1 sample) 83"("B/AO1 (Pin 4)"=0.0) -> ()  [unwired: 1 in, 1 out]
                          n238 = Subtract(x=w2649, y=w2646) -> (x-y=w2647:dbl)
                          n239 = xnode "Analog output (1 sample) 80"("A/AO0 (Pin 2)"=w2651) -> ()  [unwired: 1 in, 1 out]
                          n240 = xnode "Analog output (1 sample) 82"("B/AO0 (Pin 2)"=w2651) -> ()  [unwired: 1 in, 1 out]
                          n241 = Greater Or Equal?(x=w2647, y="tijdsinterval 7") -> (x >= y?=w2645:bool)
                        }
                      }
                      frame #4 {
                        n242 = global read "Global.vi" "Array"() -> (w2802:dbl[])
                        n243 = Delete From Array(array=w2802, length=1, index=0) -> (array with subset deleted=w2801:dbl[])  [unwired: 1 out]
                        n244 = global write "Global.vi" "Array"(w2801) -> ()
                      }
                    }
                  }
                }
                n245 = Equal?(x=w2175, y=2) -> (x = y?=w2178:bool)
                n246 = Equal?(x=1, y=w2175) -> (x = y?=w2179:bool)
                n247 = case shown="True" w2178 {
                  frame False {
                  }
                  frame True {
                    n248 = flat-sequence {
                      frame #0 {
                        w3429 = 0.0
                        # "motor  stilleggen"
                        n249 = xnode "Analog output (1 sample) 55"("A/AO1 (Pin 4)"=w3429) -> ()  [unwired: 1 in, 1 out]
                        n250 = xnode "Analog output (1 sample) 7"("B/AO0 (Pin 2)"=w3429) -> ()  [unwired: 1 in, 1 out]
                        n251 = xnode "Analog output (1 sample) 8"("A/AO0 (Pin 2)"=w3429) -> ()  [unwired: 1 in, 1 out]
                        n252 = xnode "Analog output (1 sample) 56"("B/AO1 (Pin 4)"=w3429) -> ()  [unwired: 1 in, 1 out]
                      }
                      frame #1 {
                        n253 = Get Date/Time In Seconds() -> (seconds since 1Jan1904=w3578:timestamp)
                        n254 = while {
                          tunnel: w3578 -> [w3583]
                          stop <- w3579 stop-if-true
                          w3581 = 5.0
                          # "rechtdoor"
                          # "kleursensor"
                          n255 = xnode "Analog output (1 sample) 9"("A/AO0 (Pin 2)"=w3581) -> ()  [unwired: 1 in, 1 out]
                          n256 = xnode "Analog output (1 sample) 63"("B/AO0 (Pin 2)"=w3581) -> ()  [unwired: 1 in, 1 out]
                          n257 = Get Date/Time In Seconds() -> (seconds since 1Jan1904=w3584:timestamp)
                          n258 = xnode "Analog output (1 sample) 64"("B/AO1 (Pin 4)"=0.0) -> ()  [unwired: 1 in, 1 out]
                          n259 = xnode "Analog output (1 sample) 10"("A/AO1 (Pin 4)"=0.0) -> ()  [unwired: 1 in, 1 out]
                          n260 = Subtract(x=w3584, y=w3583) -> (x-y=w3586:dbl)
                          n261 = Greater Or Equal?(x=w3586, y="tijdsinterval 5") -> (x >= y?=w3579:bool)
                        }
                      }
                      frame #2 {
                        n262 = global read "Global.vi" "Array"() -> (w3736:dbl[])
                        n263 = Delete From Array(array=w3736, length=1, index=0) -> (array with subset deleted=w3735:dbl[])  [unwired: 1 out]
                        n264 = global write "Global.vi" "Array"(w3735) -> ()
                      }
                    }
                  }
                }
                n265 = case shown="True" w2179 {
                  frame False {
                  }
                  frame True {
                    n266 = flat-sequence {
                      frame #0 {
                        w2805 = 0.0
                        # "motor  stilleggen"
                        n267 = xnode "Analog output (1 sample)"("A/AO1 (Pin 4)"=w2805) -> ()  [unwired: 1 in, 1 out]
                        n268 = xnode "Analog output (1 sample) 54"("B/AO1 (Pin 4)"=w2805) -> ()  [unwired: 1 in, 1 out]
                        n269 = xnode "Analog output (1 sample) 53"("A/AO0 (Pin 2)"=w2805) -> ()  [unwired: 1 in, 1 out]
                        n270 = xnode "Analog output (1 sample) 2"("B/AO0 (Pin 2)"=w2805) -> ()  [unwired: 1 in, 1 out]
                      }
                      frame #1 {
                        n271 = Get Date/Time In Seconds() -> (seconds since 1Jan1904=w2954:timestamp)
                        n272 = while {
                          tunnel: w2954 -> [w2958]
                          stop <- w2955 stop-if-true
                          w2957 = 0.0
                          w2956 = 5.0
                          # "kleursensor"
                          n273 = Get Date/Time In Seconds() -> (seconds since 1Jan1904=w2959:timestamp)
                          n274 = Subtract(x=w2959, y=w2958) -> (x-y=w2961:dbl)
                          n275 = xnode "Analog output (1 sample) 13"("A/AO1 (Pin 4)"=w2957) -> ()  [unwired: 1 in, 1 out]
                          n276 = xnode "Analog output (1 sample) 50"("B/AO1 (Pin 4)"=w2957) -> ()  [unwired: 1 in, 1 out]
                          n277 = xnode "Analog output (1 sample) 4"("A/AO0 (Pin 2)"=w2956) -> ()  [unwired: 1 in, 1 out]
                          n278 = xnode "Analog output (1 sample) 49"("B/AO0 (Pin 2)"=w2956) -> ()  [unwired: 1 in, 1 out]
                          n279 = Greater Or Equal?(x=w2961, y="tijdsinterval 2") -> (x >= y?=w2955:bool)
                        }
                      }
                      frame #2 {
                        n280 = Get Date/Time In Seconds() -> (seconds since 1Jan1904=w3110:timestamp)
                        n281 = while {
                          tunnel: w3110 -> [w3113]
                          stop <- w3112 stop-if-true
                          # "90 graden draaien naar links"
                          n282 = Get Date/Time In Seconds() -> (seconds since 1Jan1904=w3116:timestamp)
                          n283 = xnode "Analog output (1 sample) 60"("A/AO1 (Pin 4)"=0.0) -> ()  [unwired: 1 in, 1 out]
                          n284 = xnode "Analog output (1 sample) 62"("B/AO1 (Pin 4)"=0.0) -> ()  [unwired: 1 in, 1 out]
                          n285 = xnode "Analog output (1 sample) 61"("B/AO0 (Pin 2)"=0.0) -> ()  [unwired: 1 in, 1 out]
                          n286 = xnode "Analog output (1 sample) 59"("A/AO0 (Pin 2)"=5.0) -> ()  [unwired: 1 in, 1 out]
                          n287 = Subtract(x=w3116, y=w3113) -> (x-y=w3114:dbl)
                          n288 = Greater Or Equal?(x=w3114, y="tijdsinterval 3") -> (x >= y?=w3112:bool)
                        }
                      }
                      frame #3 {
                        n289 = Get Date/Time In Seconds() -> (seconds since 1Jan1904=w3268:timestamp)
                        n290 = while {
                          tunnel: w3268 -> [w3270]
                          stop <- w3269 stop-if-true
                          w3275 = 5.0
                          n291 = Get Date/Time In Seconds() -> (seconds since 1Jan1904=w3273:timestamp)
                          n292 = xnode "Analog output (1 sample) 73"("A/AO1 (Pin 4)"=0.0) -> ()  [unwired: 1 in, 1 out]
                          n293 = xnode "Analog output (1 sample) 51"("B/AO1 (Pin 4)"=0.0) -> ()  [unwired: 1 in, 1 out]
                          n294 = Subtract(x=w3273, y=w3270) -> (x-y=w3271:dbl)
                          n295 = xnode "Analog output (1 sample) 74"("A/AO0 (Pin 2)"=w3275) -> ()  [unwired: 1 in, 1 out]
                          n296 = xnode "Analog output (1 sample) 52"("B/AO0 (Pin 2)"=w3275) -> ()  [unwired: 1 in, 1 out]
                          n297 = Greater Or Equal?(x=w3271, y="tijdsinterval 4") -> (x >= y?=w3269:bool)
                        }
                      }
                      frame #4 {
                        n298 = global read "Global.vi" "Array"() -> (w3426:dbl[])
                        n299 = Delete From Array(array=w3426, length=1, index=0) -> (array with subset deleted=w3425:dbl[])  [unwired: 1 out]
                        n300 = global write "Global.vi" "Array"(w3425) -> ()
                      }
                    }
                  }
                }
              }
            }
          }
        }
        n301 = xnode "Digital input (1 sample)"() -> ("A/DIO1 (Pin 13)"=w40:bool)  [unwired: 1 in, 1 out]
        "A/DIO1 (Pin 13)" <- w40
        n302 = case shown="False" w40 {
          frame False {
            (unwired) TRUE
          }
          frame True {
            (unwired) FALSE
          }
        }
      }
      frame True {
        # "Manueel bedienen"
        n303 = case shown="True" "links draaien" {
          frame False {
          }
          frame True {
            n304 = xnode "Analog output  rechts 4"("B/AO1 (Pin 4)"=0.0) -> ()  [unwired: 1 in, 1 out]
            n305 = xnode "Analog output  rechts 2"("A/AO1 (Pin 4)"=0.0) -> ()  [unwired: 1 in, 1 out]
            n306 = xnode "Analog output  rechts 3"("B/AO0 (Pin 2)"=0.0) -> ()  [unwired: 1 in, 1 out]
            n307 = xnode "Analog output  links 2"("A/AO0 (Pin 2)"=5.0) -> ()  [unwired: 1 in, 1 out]
          }
        }
        n308 = case shown="True" "rechts draaien" {
          frame False {
          }
          frame True {
            n309 = xnode "Analog output  rechts 6"("B/AO1 (Pin 4)"=0.0) -> ()  [unwired: 1 in, 1 out]
            n310 = xnode "Analog output  rechts"("A/AO1 (Pin 4)"=0.0) -> ()  [unwired: 1 in, 1 out]
            n311 = xnode "Analog output  rechts 5"("B/AO0 (Pin 2)"=5.0) -> ()  [unwired: 1 in, 1 out]
            n312 = xnode "Analog output  links"("A/AO0 (Pin 2)"=0.0) -> ()  [unwired: 1 in, 1 out]
          }
        }
        n313 = case shown="True" "stoppen" {
          frame False {
          }
          frame True {
            w3782 = 0.0
            n314 = xnode "Analog output 17"("A/AO0 (Pin 2)"=w3782) -> ()  [unwired: 1 in, 1 out]
            n315 = xnode "Analog output 16"("A/AO1 (Pin 4)"=w3782) -> ()  [unwired: 1 in, 1 out]
            n316 = xnode "Analog output 15"("B/AO0 (Pin 2)"=w3782) -> ()  [unwired: 1 in, 1 out]
            n317 = xnode "Analog output 14"("B/AO1 (Pin 4)"=w3782) -> ()  [unwired: 1 in, 1 out]
          }
        }
        n318 = case shown="True" "links draaien achteruit" {
          frame False {
          }
          frame True {
            n319 = xnode "Analog output 7"("B/AO0 (Pin 2)"=0.0) -> ()  [unwired: 1 in, 1 out]
            n320 = xnode "Analog output 6"("B/AO1 (Pin 4)"=0.0) -> ()  [unwired: 1 in, 1 out]
            n321 = xnode "Analog output 8"("A/AO1 (Pin 4)"=5.0) -> ()  [unwired: 1 in, 1 out]
            n322 = xnode "Analog output 9"("A/AO0 (Pin 2)"=0.0) -> ()  [unwired: 1 in, 1 out]
          }
        }
        n323 = case shown="True" "rechts draaien achteruit" {
          frame False {
          }
          frame True {
            n324 = xnode "Analog output 11"("B/AO0 (Pin 2)"=0.0) -> ()  [unwired: 1 in, 1 out]
            n325 = xnode "Analog output 10"("B/AO1 (Pin 4)"=5.0) -> ()  [unwired: 1 in, 1 out]
            n326 = xnode "Analog output 12"("A/AO1 (Pin 4)"=0.0) -> ()  [unwired: 1 in, 1 out]
            n327 = xnode "Analog output 13"("A/AO0 (Pin 2)"=0.0) -> ()  [unwired: 1 in, 1 out]
          }
        }
        n328 = case shown="True" "voorwaarts" {
          tunnel: "snelheid" -> [_ w4689]
          frame False {
          }
          frame True {
            w4690 = 0.0
            n329 = xnode "Analog output (1 sample) 16"("A/AO0 (Pin 2)"=w4689) -> ()  [unwired: 1 in, 1 out]
            n330 = xnode "Analog output (1 sample) 15"("B/AO0 (Pin 2)"=w4689) -> ()  [unwired: 1 in, 1 out]
            n331 = xnode "Analog output 3"("A/AO1 (Pin 4)"=w4690) -> ()  [unwired: 1 in, 1 out]
            n332 = xnode "Analog output 2"("B/AO1 (Pin 4)"=w4690) -> ()  [unwired: 1 in, 1 out]
          }
        }
        n333 = case shown="True" "achterwaarts" {
          tunnel: "snelheid" -> [_ w4539]
          frame False {
          }
          frame True {
            w4540 = 0.0
            n334 = xnode "Analog output (1 sample) 17"("A/AO1 (Pin 4)"=w4539) -> ()  [unwired: 1 in, 1 out]
            n335 = xnode "Analog output 5"("B/AO1 (Pin 4)"=w4539) -> ()  [unwired: 1 in, 1 out]
            n336 = xnode "Analog output (1 sample) 18"("A/AO0 (Pin 2)"=w4540) -> ()  [unwired: 1 in, 1 out]
            n337 = xnode "Analog output 4"("B/AO0 (Pin 2)"=w4540) -> ()  [unwired: 1 in, 1 out]
          }
        }
      }
    }
  }
